vi "Memory Benchmark.vi"(5 "Show Cache Lines (F)":bool, 7 "Show Peak Bandwidth (F)":bool, 9 "Transfers (500)":i32=500, 10 "End Size":u64=100000000 format="%.0pB", 11 "Start Size":u64=1000 format="%.0pB") -> (3 "Memory Bandwidth":cluster{"X":dbl[], "Y":dbl[]}[](graph) caption="Memory Bandwidth Plot")   [LabVIEW 2020]
uses:
  Classes/Pointer/Stop/Stop Pointer.lvclass
  Classes/Pointer/Pointer.lvclass
  UI Pointers.ctl
  Classes/Pointer/Write I32.vi
  Classes/Pointer/Read I32.vi
panel:
  out "Progress Message":string
  out "Progress":dbl(slide) scale=0.0..1.0
  out "Peak Throughput":dbl format="%.3pB/s"
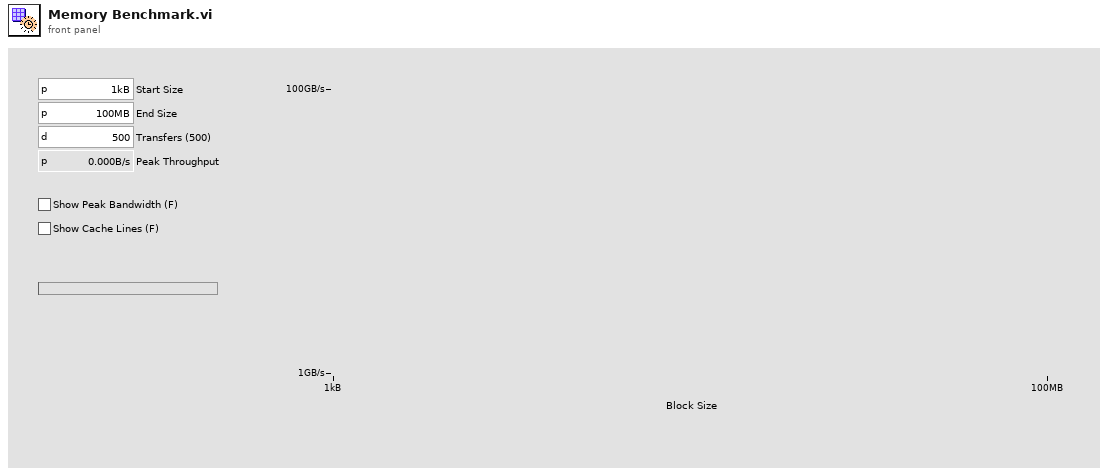
[diagram p1: front panel]
types:
  T1 = typedef "UI Pointers.ctl" = cluster{"Stop Pointer":refnum<class "Stop Pointer.lvclass">, "Iteration Pointer":refnum<class "Pointer.lvclass">}
  T2 = typedef "LVAnnotationListTypeDef.ctl" = cluster{"Name":string, "Color":u32, "Style":u8, "Point Style":u8, "Name Visible":bool, "Allow Drag":bool, "Annotation Mode":u32, "Plot":i32, "Index":i32, "Position":cluster{"X":dbl, "Y":dbl}, "X Scale":u32, "Y Scale":u32, "Show Arrow":bool, "Lock Name":bool, "Plot Area":i32, "Label Offset":cluster{"X":dbl, "Y":dbl}}[]
  T3 = cluster{"Name":string, "Color":u32, "Style":u8, "Point Style":u8, "Name Visible":bool, "Allow Drag":bool, "Annotation Mode":u32, "Plot":i32, "Index":i32, "Position":cluster{"X":dbl, "Y":dbl}, "X Scale":u32, "Y Scale":u32, "Show Arrow":bool, "Lock Name":bool, "Plot Area":i32, "Label Offset":cluster{"X":dbl, "Y":dbl}}
  T4 = cluster{"Name":string, "Color":u32, "Style":u8, "Point Style":u8, "Name Visible":bool, "Allow Drag":bool, "Annotation Mode":u32, "Plot":i32, "Index":i32, "Position":cluster{"X":dbl, "Y":dbl}, "X Scale":u32, "Y Scale":u32, "Show Arrow":bool, "Lock Name":bool, "Plot Area":i32, "Label Offset":cluster{"X":dbl, "Y":dbl}}[]
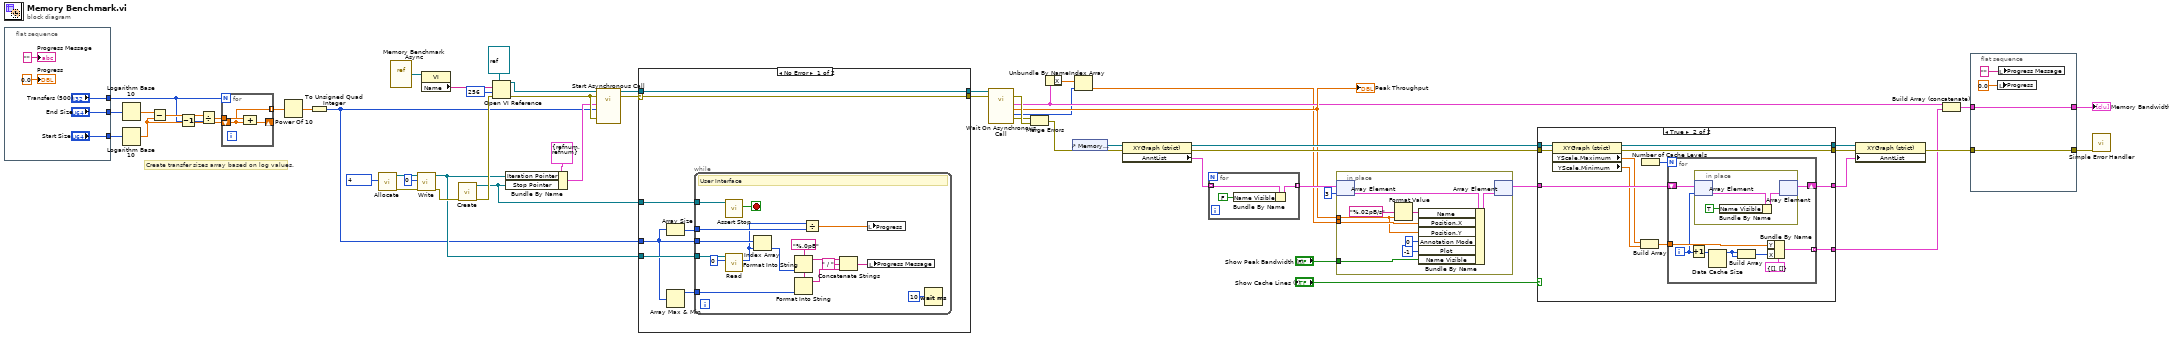
[diagram p0: block diagram]
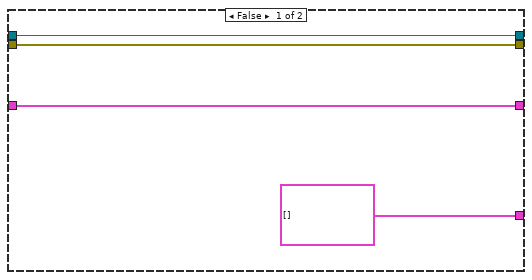
[diagram p3: hidden frame]
diagram:
  # "Create transfer sizes array based on log values."
  n1 = flat-sequence {
    tunnel: ["Start Size"] -> w55
    tunnel: ["End Size"] -> w54
    tunnel: ["Transfers (500)"] -> w49
    frame #0 {
      "Progress" <- 0.0 ("Progress")
      "Progress Message" <- "" ("String")
    }
  }
  n2 = Logarithm Base 10(1:w54) -> (0:w53:dbl)
  n3 = Logarithm Base 10(1:w55) -> (0:w50:dbl)
  n4 = Subtract(x=w53, y=w50) -> (x-y=w52:dbl)
  n5 = Decrement(x=w49) -> (x-1=w48:i32)
  n6 = Divide(x=w52, y=w48) -> (x/y=w51:dbl)
  n7 = for {
    N: w49 -> [_]
    tunnel: w51 -> [w64]
    shift-right: [w63] -> _
    shift-left: w50 -> [w62]
    tunnel: [w62] -> w47 mode=indexing
    n8 = Compound Arithmetic op=ADD(w64, w62) -> (w63:dbl)
  }
  n9 = Power Of 10(x=w47) -> (10^x=w46:dbl[])
  n10 = To Unsigned Quad Integer(1:w46) -> (0:w3:u64[])
  n11 = call "Allocate.vi"("size"=u64 4) -> ("error out"=w32:errorcluster, "Pointer out"=w30:refnum<class "Pointer.lvclass">)  [unwired: 9 in]
  n12 = vi-ref "Memory Benchmark Async.vi"() -> (w22:refnum<vi>)
  n13 = call-poly "Write.vi"("error in (no error)"=w32, "value"=0, "Pointer in"=w30) -> ("error out"=w29:errorcluster, "Pointer out"=w13:refnum<class "Pointer.lvclass">)  [unwired: 5 in, 2 out]
  n14 = property class="VI"(reference=w22) -> ("Name"=w21:string)  [unwired: 1 in, 2 out]
  n15 = call "Create.vi"("error in (no error)"=w29) -> ("error out"=w15:errorcluster, "Stop Pointer"=w14:refnum<class "Stop Pointer.lvclass">)  [unwired: 9 in]
  n16 = Open VI Reference(type specifier VI Refnum (for type only)=refnum<vi> refnum, vi path=w21, options=256, error in (no error)=w15) -> (vi reference=w20:refnum<vi>, error out=w12:errorcluster)  [unwired: 2 in]
  n17 = Bundle By Name(cluster=T1 {"Stop Pointer"=refnum, "Iteration Pointer"=refnum} ("UI Pointers"), "Iteration Pointer"=w13, "Stop Pointer"=w14) -> (w11:T1)
  n18 = call-by-ref "Start Asynchronous Call"(reference=w20, error in=w12, 8:"error in (no error)"=w12, "copy sizes"=w3, "UI Pointers"=w11) -> (reference out=w6:refnum<vi>, error out=w10:errorcluster)  [unwired: 5 in, 4 out]
  n19 = case shown="No Error" w10 {
    selector: w10 -> [w68 w88]
    tunnel: w14 -> [w70 _]
    tunnel: w13 -> [w69 _]
    tunnel: w3 -> [w65 _]
    tunnel: [w68 w88] -> w9
    tunnel: w6 -> [w67 w89]
    tunnel: [w67 w89] -> w5
    frame No Error {
      n20 = Array Size(array=w65) -> (size(s)=w71:i32)
      n21 = Array Max & Min(array=w65) -> (max value=w66:u64)  [unwired: 3 out]
      n22 = while {
        tunnel: w70 -> [w87]
        tunnel: w69 -> [w84]
        tunnel: w65 -> [w82]
        tunnel: w66 -> [w79]
        tunnel: w71 -> [w73]
        stop <- w86 stop-if-true
        w80 = "%.0pB" ("format string")
        # "User Interface"
        n23 = call "Assert Stop.vi"("Stop Pointer in"=w87) -> ("stop?"=w86:bool)  [unwired: 8 in, 2 out]
        n24 = call-poly "Read.vi"("value in"=0, "Pointer in"=w84) -> ("value out"=w72:i32)  [unwired: 6 in, 3 out]
        n25 = Index Array(array=w82, index=w72) -> (element=w78:u64)
        n26 = Format Into String(format string=w80, w78) -> (resulting string=w77:string)  [unwired: 2 in, 1 out]
        n27 = Format Into String(format string=w80, w79) -> (resulting string=w76:string)  [unwired: 2 in, 1 out]
        n28 = Divide(x=w72, y=w73) -> (x/y=w81:dbl)
        n29 = Concatenate Strings(w77, " / " ("string"), w76) -> (w74:string)
        n30 = local write "Progress"(w81) -> ()
        n31 = local write "Progress Message"(w74) -> ()
        n32 = Wait (ms)(milliseconds to wait=u32 10) -> ()  [unwired: 1 out]
      }
    }
    frame Error {
    }
  }
  n33 = call-by-ref "Wait On Asynchronous Call"(reference=w5, error in=w9) -> (error out=w56:errorcluster, 0:"error out"=w8:errorcluster, "peak index"=w2:i32, "peak throughput"=w19:dbl, "results"=w17:cluster{"X":dbl[], "Y":dbl[]})  [unwired: 8 in, 1 out]
  "Peak Throughput" <- w19
  n34 = Merge Errors(w8, w56) -> (w7:errorcluster)
  n35 = Unbundle By Name(w17) -> ("X"=w18:dbl[])
  n36 = control-ref of="Memory Bandwidth"() -> (w42:refnum<vi>)
  n37 = Index Array(array=w18, index=w2) -> (element=w1:dbl)
  n38 = property class="XYGraph (strict)"(reference=w42, error in=w7) -> (reference out=w37:refnum<vi>, error out=w38:errorcluster, "AnntList"=w41:T2)
  n39 = for {
    tunnel: w41 -> [w91] mode=indexing
    tunnel: [w90] -> w39 mode=indexing
    n40 = Bundle By Name(cluster=w91, "Name Visible"=FALSE) -> (w90:T3)
  }
  n41 = in-place {
    in-place-border: w19 -> [w93]
    in-place-border: w1 -> [w97]
    in-place-border: "Show Peak Bandwidth (F)" -> [w94]
    n42 = in-place-array #1(w39, 3) -> (w101:T3)
    n43 = Format Value(format string="%.02pB/s", value (0)=w93) -> (output string=w99:string)  [unwired: 1 in]
    n44 = Bundle By Name(cluster=w101, "Name"=w99, "Position.X"=w97, "Position.Y"=w93, "Annotation Mode"=u32 0, "Plot"=-1, "Name Visible"=w94) -> (w98:T3)
    n45 = in-place-array #1(w98) -> (w43:T4)  [unwired: 1 out]
  }
  n46 = case shown="True" "Show Cache Lines (F)" {
    tunnel: [cluster{"X":dbl[], "Y":dbl[]}[] [] w114] -> w25
    tunnel: w37 -> [w102 w113]
    tunnel: w43 -> [w103 w112]
    tunnel: w38 -> [w104 w111]
    tunnel: [w104 w108] -> w36
    tunnel: [w102 w107] -> w35
    tunnel: [w103 w106] -> w34
    frame False {
    }
    frame True {
      n47 = property class="XYGraph (strict)"(reference=w113, error in=w111) -> (reference out=w107:refnum<vi>, error out=w108:errorcluster, "YScale.Maximum"=w110:dbl, "YScale.Minimum"=w109:dbl)
      n48 = Build Array(w110, w109) -> (w115:dbl[])
      n49 = Number of Cache Levels() -> (w116:i32)
      n50 = for {
        N: w116 -> [_]
        tunnel: w115 -> [w121]
        tunnel: [w120] -> w114 mode=indexing
        shift-right: [w118] -> w106
        shift-left: w112 -> [w119]
        i -> [w117]
        n51 = Increment(x=w117) -> (x+1=w125:i32)
        n52 = in-place {
          n53 = in-place-array #2(w119, w117) -> (w128:T3)
          n54 = Bundle By Name(cluster=w128, "Name Visible"=TRUE) -> (w127:T3)
          n55 = in-place-array #2(w127) -> (w118:T4)  [unwired: 1 out]
        }
        n56 = Data Cache Size(0:w125) -> (4:w123:i32)  [unwired: 1 out]
        n57 = Build Array(w123, w123) -> (w122:i32[])
        n58 = Bundle By Name(cluster=cluster{"X":dbl[], "Y":dbl[]} {"X"=[], "Y"=[]}, "Y"=w121, "X"=w122) -> (w120:cluster{"X":dbl[], "Y":dbl[]})
      }
    }
  }
  n59 = property class="XYGraph (strict)"(reference=w35, error in=w36, "AnntList"=w34) -> (error out=w26:errorcluster)  [unwired: 1 out]
  n60 = Build Array (concatenate)(w17, w25) -> (w28:cluster{"X":dbl[], "Y":dbl[]}[])
  n61 = flat-sequence {
    tunnel: w28 -> [w130]
    tunnel: [w130] -> w27
    tunnel: w26 -> [w129]
    tunnel: [w129] -> w24
    frame #0 {
      n62 = local write "Progress"(0.0 ("Progress")) -> ()
      n63 = local write "Progress Message"("" ("String")) -> ()
    }
  }
  n64 = call <vilib>:"Simple Error Handler.vi"("error in (no error)"=w24) -> ()  [unwired: 4 in, 5 out]
  "Memory Bandwidth" <- w27
